vi "Protocol.Convert Signals to Frame by ID.vi"(8 "error in (no error)":errorcluster, 9 "ID":u32, 10 "RequestDataTable":refnum<k33>, 11 "Data LUT":variant) -> (0 "error out":errorcluster, 2 "Found?":bool, 3 "Frame":T1 {"Identifier" format="%08x"})   [LabVIEW 2015, in "J1939 Addon Engine.lvlib"]
uses:
  J1939 Addon Engine.lvlib
  Shared/J1939 Utilities/Types/CAN Outgoing Message Cluster.ctl
  Shared/Types/Outgoing Frame Settings.ctl
  Shared/Types/Outgoing Event Trigger Types.ctl
  <vilib>/xnet/xnet.llb/XNET Convert (Signal to Frame CAN).vi
  <vilib>/xnet/xnet.llb/XNET Create Session (Conversion).vi
  Shared/J1939 Utilities/J1939 Utilities.lvlib
  Shared/J1939 Addon Shared.lvlib
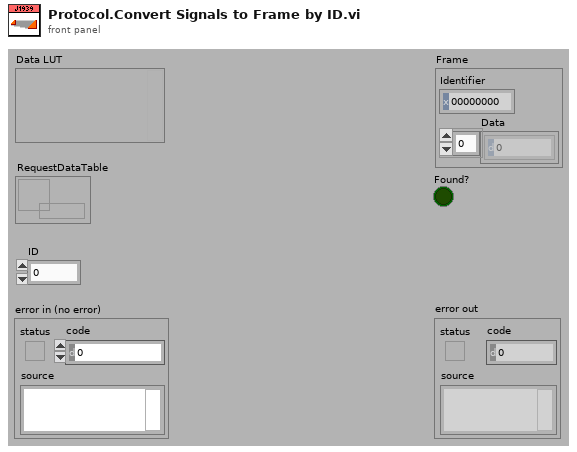
[diagram p1: front panel]
types:
  T1 = typedef "J1939 Addon Shared.lvlib/J1939 Utilities.lvlib/CAN Outgoing Message Cluster.ctl" = cluster{"Identifier":u32, "Data":u8[]}
  T2 = typedef "J1939 Addon Shared.lvlib/Outgoing Frame Settings.ctl" = cluster{"Signals":string[], "Channel Array Position":cluster{"Offset":u32, "Length":u32}, "PGN":u32, "Cyclic?":bool, "Disable?":bool, "Disable.Index":i32, "Trigger":T3, "Trigger.Index":i32}
  T3 = typedef "J1939 Addon Shared.lvlib/Outgoing Event Trigger Types.ctl" = enum16{"Channel value change", "Trigger channel (not zero)", "Channel value change or trigger channel (not zero)", "Trigger channel (any value change)", "Channel value change or trigger channel (any value change)"}
  T4 = typedef "XNET Frame CAN.ctl" = cluster{"timestamp":timestamp, "payload":u8[], "identifier":u32, "type":T5, "extended?":bool, "echo?":bool}
  T5 = typedef "XNET Frame Type CAN.ctl" = u8
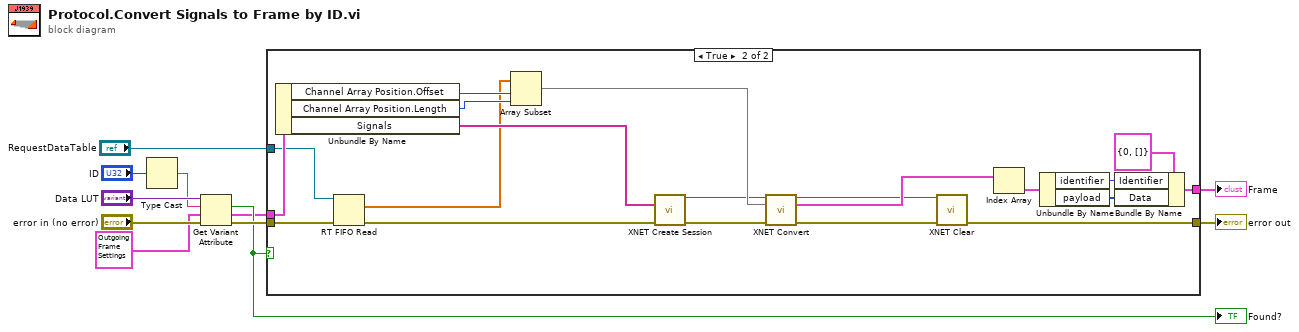
[diagram p0: block diagram]
diagram:
  n1 = Type Cast(x="ID") -> (*(type *) &x=w5:string)  [unwired: 1 in]
  n2 = Get Variant Attribute(Variant="Data LUT", name=w5, default value (empty Variant)=T2 {"Signals"=[], "Channel Array Position"={"Offset"=0, "Length"=0}, "PGN"=0, "Cyclic?"=FALSE, "Disable?"=FALSE, "Disable.Index"=0, "Trigger"=enum."Channel value change", "Trigger.Index"=0} ("Frame"), error in="error in (no error)") -> (found=w3:bool, value=w1:T2, error out=w8:errorcluster)  [unwired: 1 out]
  "Found?" <- w3
  n3 = case shown="True" w3 {
    tunnel: w1 -> [_ w32]
    tunnel: w8 -> [w12 w15]
    tunnel: [w12 w17] -> w11
    tunnel: [_ w30] -> w10
    tunnel: "RequestDataTable" -> [_ w16]
    frame False {
    }
    frame True {
      n4 = Unbundle By Name(w32) -> ("Channel Array Position.Offset"=w29:u32, "Channel Array Position.Length"=w28:u32, "Signals"=w26:string[])
      n5 = RT FIFO Read(0:w16, 3:w15) -> (9:w13:dbl[], 11:w14:errorcluster)  [unwired: 2 in, 3 out]
      n6 = Array Subset(array=w13, index=w29, length=w28) -> (w25:dbl[])
      n7 = call-poly <vilib>:"XNET Create Session.vi"("signal list"=w26, "error in (no error)"=w14) -> ("session out"=w24:refnum<k21>, "error out"=w27:errorcluster)  [unwired: 12 in]
      n8 = call-poly <vilib>:"XNET Convert.vi"("session in"=w24, "signal data"=w25, "error in (no error)"=w27) -> ("session out"=w19:refnum<k21>, "frame data"=w23:T4[], "error out"=w18:errorcluster)  [unwired: 9 in, 1 out]
      n9 = call <vilib>:"XNET Clear.vi"("session in"=w19, "error in (no error)"=w18) -> ("error out"=w17:errorcluster)  [unwired: 13 in]
      n10 = Index Array(array=w23) -> (element=w22:T4)  [unwired: 1 in]
      n11 = Unbundle By Name(w22) -> ("identifier"=w21:u32, "payload"=w20:u8[])
      n12 = Bundle By Name(cluster=T1 {"Identifier"=0, "Data"=[]} ("element"), "Identifier"=w21, "Data"=w20) -> (w30:T1)
    }
  }
  "error out" <- w11
  "Frame" <- w10
